vi "Set ObjFlags.vi"(8 "error in (no error)":errorcluster, 10 "ObjFlags":u32, 11 "OD Entry in":refnum<class "OD Entry.lvclass">) -> (0 "error out":errorcluster, 3 "OD Entry out":refnum<class "OD Entry.lvclass">)   [LabVIEW 2024, in "OD Entry.lvclass"]
uses:
  OD Entry.lvclass
  OD Entry.lvclass/OD Entry.ctl
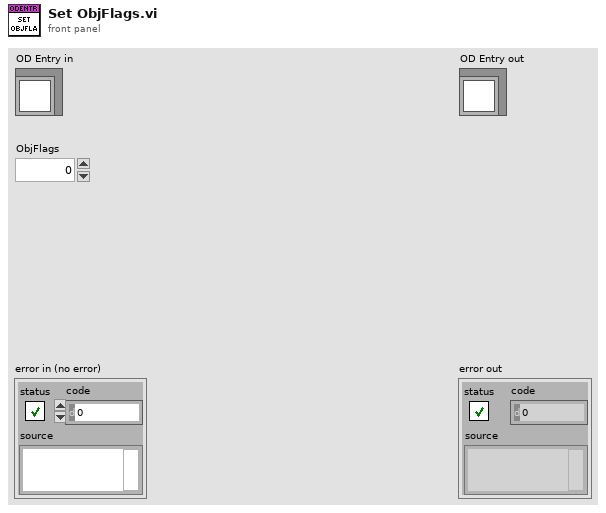
[diagram p1: front panel]
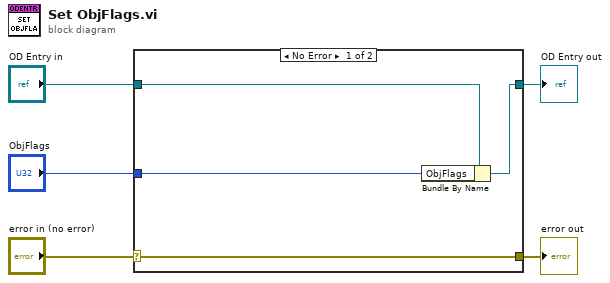
[diagram p0: block diagram]
diagram:
  n1 = case shown="No Error" "error in (no error)" {
    selector: "error in (no error)" -> [w9 w10]
    tunnel: [w9 w10] -> w4
    tunnel: [w7 w11] -> w2
    tunnel: "OD Entry in" -> [w8 w11]
    tunnel: "ObjFlags" -> [w6 _]
    frame No Error {
      n2 = Bundle By Name(cluster=w8, "ObjFlags"=w6) -> (w7:refnum<class "OD Entry.lvclass">)
    }
    frame Error {
    }
  }
  "error out" <- w4
  "OD Entry out" <- w2
